vi "Configure Trigger.vi"(0 "VISA resource name":refnum<visa-resource-name>, 1 "Enable Trigger Auto Delay (F: Disable)":bool, 2 "Enable Trigger Bypass (F: Disable)":bool, 5 "Trigger Source (0: Immediate)":u16(ring) items=["Immediate", "Tlink"], 7 "Trigger Loop Count (1)":i32=1, 9 "Trigger Delay (0 s)":dbl, 11 "error in (no error)":errorcluster) -> (4 "VISA resource name out":refnum<visa-resource-name>, 15 "error out":errorcluster)   [LabVIEW 2020, in "Keithley 648X Series.lvlib"]
doc: "Configures the event detection of the trigger layer."
uses:
  <instrlib>/Keithley 648X Series/Keithley 648X Series.lvlib
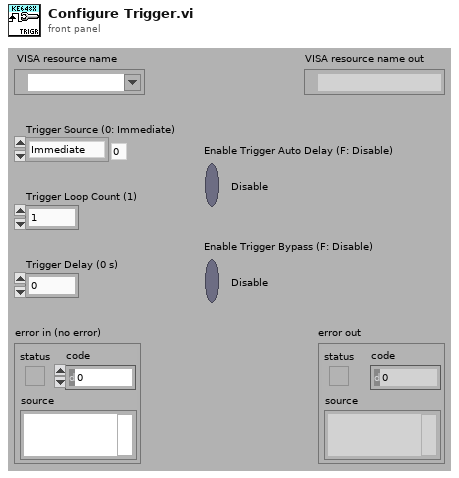
[diagram p1: front panel]
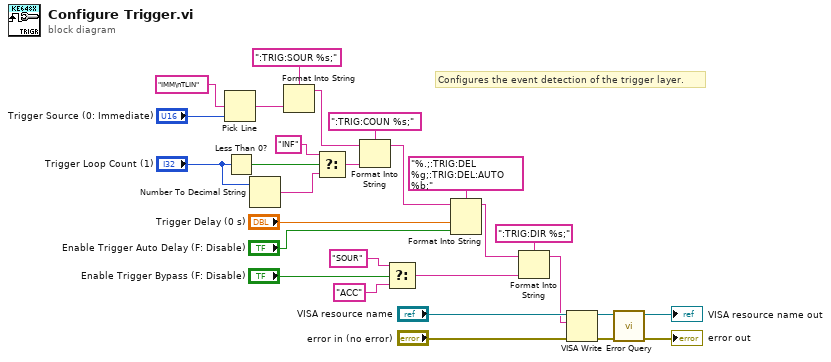
[diagram p0: block diagram]
diagram:
  # "Configures the event detection of the trigger layer."
  n1 = Pick Line(multi-line string="IMM\nTLIN", line index="Trigger Source (0: Immediate)") -> (output string=w20:string)  [unwired: 1 in]
  n2 = Less Than 0?(x="Trigger Loop Count (1)") -> (x < 0?=w17:bool)
  n3 = Number To Decimal String(number="Trigger Loop Count (1)") -> (decimal integer string=w16:string)  [unwired: 1 in]
  n4 = Format Into String(format string=":TRIG:SOUR %s;", w20) -> (resulting string=w12:string)  [unwired: 2 in, 1 out]
  n5 = Select(t="INF", s=w17, f=w16) -> (s? t:f=w14:string)
  n6 = Format Into String(format string=":TRIG:COUN %s;", initial string=w12, w14) -> (resulting string=w10:string)  [unwired: 1 in, 1 out]
  n7 = Select(t="SOUR", s="Enable Trigger Bypass (F: Disable)", f="ACC" ("t")) -> (s? t:f=w3:string)
  n8 = Format Into String(format string="%.;:TRIG:DEL %g;:TRIG:DEL:AUTO %b;", initial string=w10, "Trigger Delay (0 s)", "Enable Trigger Auto Delay (F: Disable)") -> (resulting string=w2:string)  [unwired: 1 in, 1 out]
  n9 = Format Into String(format string=":TRIG:DIR %s;", initial string=w2, w3) -> (resulting string=w1:string)  [unwired: 1 in, 1 out]
  n10 = VISA Write(VISA resource name="VISA resource name", write buffer=w1, error in (no error)="error in (no error)") -> (VISA resource name out=w24:refnum<visa-resource-name>, error out=w23:errorcluster)  [unwired: 1 out]
  n11 = call <instrlib>:"Error Query.vi"("error in (no error)"=w23, "VISA resource name"=w24) -> ("error out"=→"error out":errorcluster, "VISA resource name out"=→"VISA resource name out":refnum<visa-resource-name>)  [unwired: 6 in, 2 out]
